vi "New.vi"(8 "Error In":errorcluster) -> (0 "Error Out":errorcluster, 3 "Root":refnum<class "Root.lvclass">)   [LabVIEW 2018, in "Toolkit.lvlib" / "Nodes.lvlib" / "Root.lvclass"]
uses:
  Root.lvclass
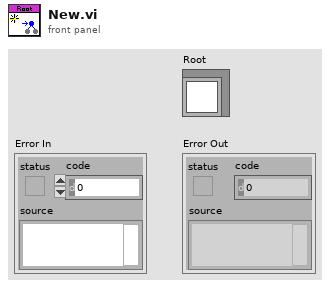
[diagram p1: front panel]
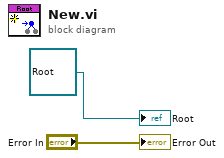
[diagram p0: block diagram]
diagram:
  "Error Out" <- "Error In"
  "Root" <- refnum<class "Root.lvclass"> refnum ("Toolkit.lvlib:Nodes.lvlib:Root.lvclass")
